vi "DataFormating.vi"(8 "Voltage":dbl format="%#_6f", 11 "Data from Sensor":T2) -> (1 "output":T1, 2 "Tank 2":dbl format="%#_6f", 3 "Tank 1":dbl format="%#_6f")   [LabVIEW 2011]
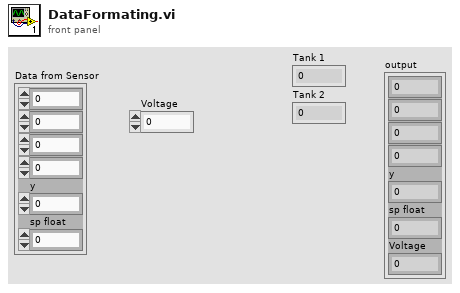
[diagram p1: front panel]
types:
  T1 = cluster{dbl, dbl, dbl, dbl, "y":dbl, "sp float":u8, "Voltage ":dbl}
  T2 = cluster{dbl, dbl, dbl, dbl, "y":dbl, "sp float":u8}
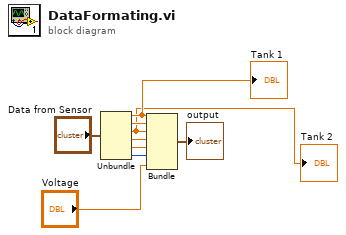
[diagram p0: block diagram]
diagram:
  n1 = Unbundle("Data from Sensor") -> (w5:dbl, w6:dbl, w2:dbl, w7:dbl, "y"=w8:dbl, "sp float"=w9:u8)
  "Tank 1" <- w5
  "Tank 2" <- w2
  n2 = Bundle(w5, w6, w2, w7, "y"=w8, "sp float"=w9, "Voltage"="Voltage") -> (→"output":T1)  [unwired: 1 in]
